vi "AcquisitionInterface3.vi"() -> ()   [LabVIEW 2025]
uses:
  <vilib>/DAQmx/read.llb/DAQmx Read (Analog 1D Wfm NChan NSamp).vi
  <vilib>/DAQmx/miscellaneous.llb/DAQmx Fill In Error Info.vi
  <vilib>/Waveform/WDTOps.llb/WDT Append Waveforms DBL.vi
panel:
  in  "Max Y value":dbl(slide) min=0.0 max=10.0 scale=0.0..10.0
  in  "frequency settings":T1={"frequency (Hz)"=1000.0, "number of samples per cycle"=50.0, "number of cycles"=1.0}
  out "file path out":path
  out "error out":errorcluster
  in  "Save to txt":bool
  in  "stop":bool
  out "data":waveform(dbl)(graph)
  in  "error in":errorcluster
  in  "physical channels":tag
  # "Pulsa este botón para que la señal medida se guarde en un archivo .txt"
  # "La señal se ha guardado en:"
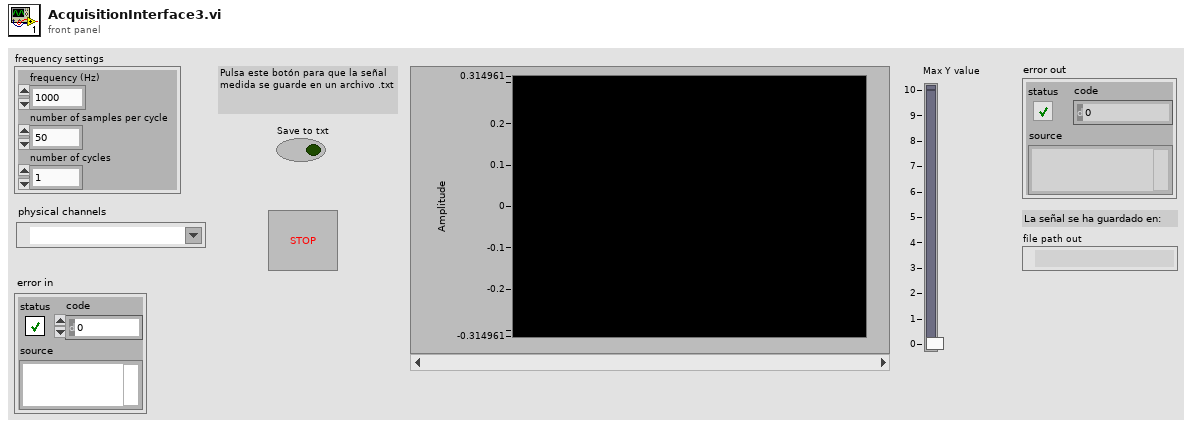
[diagram p1: front panel]
types:
  T1 = cluster{"frequency (Hz)":dbl, "number of samples per cycle":dbl, "number of cycles":dbl}
  T2 = cluster{"units":i32, "input terminal configuration":i32, "maximum value":dbl, "minimum value":dbl}
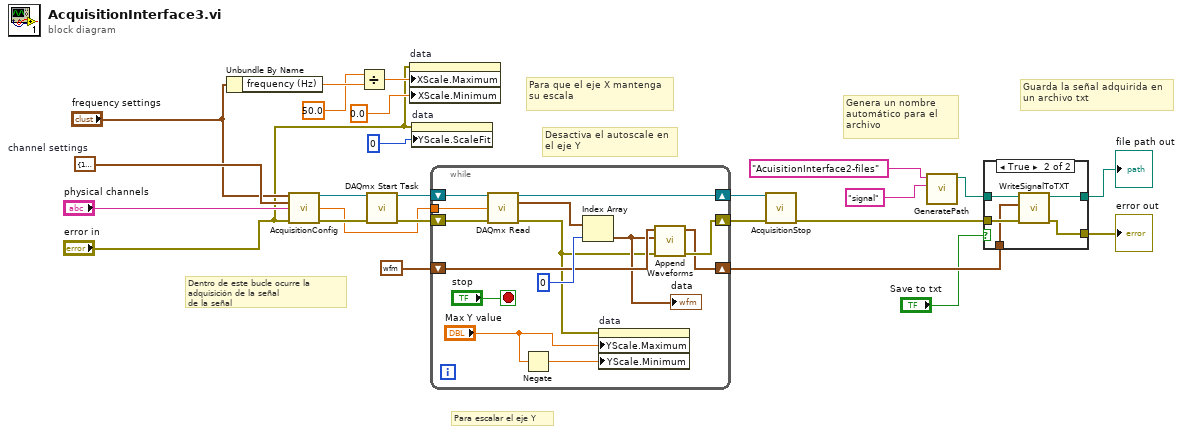
[diagram p0: block diagram]
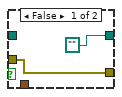
[diagram p2: hidden frame]
diagram:
  w18 = T2 {"units"=10348, "input terminal configuration"=10083, "maximum value"=1.5, "minimum value"=-1.5}  # channel settings
  # "Para escalar el eje Y"
  # "Desactiva el autoscale en el eje Y"
  # "Genera un nombre automático para el archivo"
  # "Para que el eje X mantenga su escala"
  # "Guarda la señal adquirida en\nun archivo txt"
  # "Dentro de este bucle ocurre la adquisición de la señal\nde la señal"
  n1 = Unbundle By Name("frequency settings") -> ("frequency (Hz)"=w9:dbl)
  n2 = call "AcquisitionConfig.vi"("frequency settings"="frequency settings", "channel settings"=w18, "physical channels"="physical channels", "error in"="error in") -> ("task out"=w23:refnum<k21>, "number of samples"=w17:dbl, "error out"=w24:errorcluster)  [unwired: 9 in]
  n3 = Divide(x=50.0, y=w9) -> (x/y=w7:dbl)
  n4 = call <vilib>:"DAQmx Start Task.vi"("task/channels in"=w23, "error in"=w24) -> ("task out"=w21:refnum<k21>, "error out"=w22:errorcluster)  [unwired: 12 in]
  n5 = property on="data" class="WFChart (strict)"(error in="error in", "XScale.Maximum"=w7, "XScale.Minimum"=0.0 ("X Scale.Range:Minimum")) -> ()  [unwired: 1 in, 2 out]
  n6 = property on="data" class="WFChart (strict)"(error in="error in", "YScale.ScaleFit"=u8 0 ("Y Scale.Scale Fit")) -> ()  [unwired: 1 in, 2 out]
  n7 = while {
    tunnel: w17 -> [w37]
    shift-right: [w31] -> w20
    shift-left: w22 -> [w32]
    shift-right: [w38] -> w19
    shift-left: w21 -> [w39]
    shift-right: [w29] -> w14
    shift-left: waveform(dbl) {"t0"=timestamp(0 s since 1904-01-01), "dt"=1.0, "Y"=[]} ("waveform out") -> [w33]
    stop <- "stop" stop-if-true
    n8 = call-poly <vilib>:"DAQmx Read.vi"("task/channels in"=w39, "number of samples per channel"=w37, "error in"=w32) -> ("task out"=w38:refnum<k21>, "data"=w34:waveform(dbl)[], "error out"=w28:errorcluster)  [unwired: 10 in]
    n9 = Negate(x="Max Y value") -> (-x=w27:dbl)
    n10 = Index Array(array=w34, index=0) -> (element=w30:waveform(dbl))
    "data" <- w30
    n11 = property on="data" class="WFChart (strict)"(error in=w28, "YScale.Maximum"="Max Y value", "YScale.Minimum"=w27) -> ()  [unwired: 1 in, 2 out]
    n12 = call-poly <vilib>:"Append Waveforms.vi"("error in (no error)"=w28, "waveform B"=w30, "waveform A"=w33) -> ("error out"=w31:errorcluster, "waveform out"=w29:waveform(dbl))  [unwired: 7 in]
  }
  n13 = call "AcquisitionStop.vi"("task/channels in"=w19, "error in"=w20) -> ("error out"=w15:errorcluster)  [unwired: 13 in]
  n14 = call "GeneratePath.vi"("file name (no extension)"="signal", "folder  name"="AcuisitionInterface2-files") -> ("path"=w5:path)  [unwired: 9 in]
  n15 = case shown="True" "Save to txt" {
    tunnel: w15 -> [w41 w46]
    tunnel: w14 -> [_ w45]
    tunnel: [w41 w44] -> w12
    tunnel: [path "" w43] -> w11
    tunnel: w5 -> [_ w42]
    frame False {
    }
    frame True {
      n16 = call "WriteSignalToTXT.vi"("error in"=w46, "waveform"=w45, "file path in"=w42) -> ("error out"=w44:errorcluster, "file path out"=w43:path)  [unwired: 7 in]
    }
  }
  "error out" <- w12
  "file path out" <- w11
